vi "iv-sweep-with-dpo3014.vi"(3 "Oscilloscope Address":refnum<visa-resource-name>="USB0::0x0699::0x0411::C023742::INSTR") -> (0 "Indicator of finish":bool=TRUE)   [LabVIEW 2013]
uses:
  <vilib>/Analysis/NI_AALBase.lvlib
  <vilib>/Analysis/baseanly.llb/Mean (DBL).vi
panel:
  in  "Averages":u32=1000 step=1
  out "Channel  1 Graph":dbl[](graph)
  out "Channel  2 Graph":dbl[](graph)
  in  "Cut from end":u32=1000 step=1
  in  "Cut from start":u32=1000 step=1
  in  "Sweep End (V)":dbl=2.0 min=0.002 max=10.0 step=0.001 format="%#_6p"
  in  "Sweep Start (V)":dbl min=0.002 max=10.0 step=0.001 format="%#_6p"
  in  "Sweep Func":u16(ring) items=["SIN", "SQR", "TRI", "RMP", "PLS"]
  in  "Sweep Freq":u16(ring)=15 items=["1MHz", "250kHz", "125kHz", "100kHZ", "25kHz", "10kHz", "5kHz", "2.5kHz", "1kHz", "500Hz", "250Hz", "100Hz", "50Hz", "25Hz", "10Hz", "5Hz", "2.5Hz", "1Hz", "0.5Hz", "0.25Hz"]
  in  "Yokogawa Sweep GPIB":string="18"
  out "Time Range (s)":dbl=0.02 format="%.2p"
  in  "Points per sweep":u16(ring)=1 items=["1000", "10000", "100000", "1000000", "5000000"]
  in  "Trig Delay (s)":dbl step=0.0001 format="%#_6p"
  out "Query Return":string=":ACQUIRE:STOPAFTER SEQUENCE;STATE 1;MODE AVERAGE;NUMENV INFINITE;NUMAVG 2;MAXSAMPLERATE 2.5000E+9\n"
  in  "Query":string="ACQUIRE?"
  out "Time Taken (s)":dbl=1.35 format="%.2p"
  # "If changed, run program once before real readout"
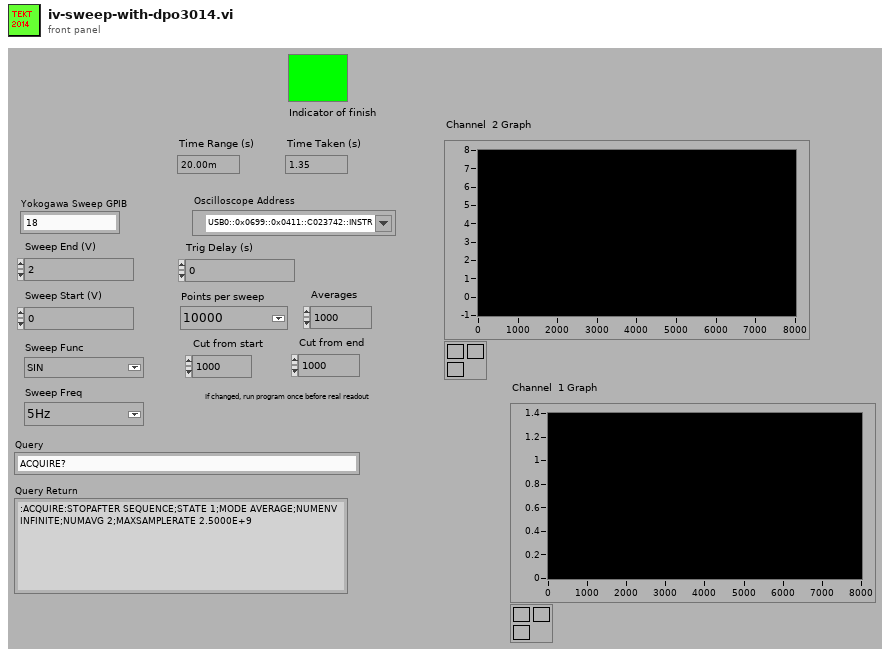
[diagram p1: front panel]
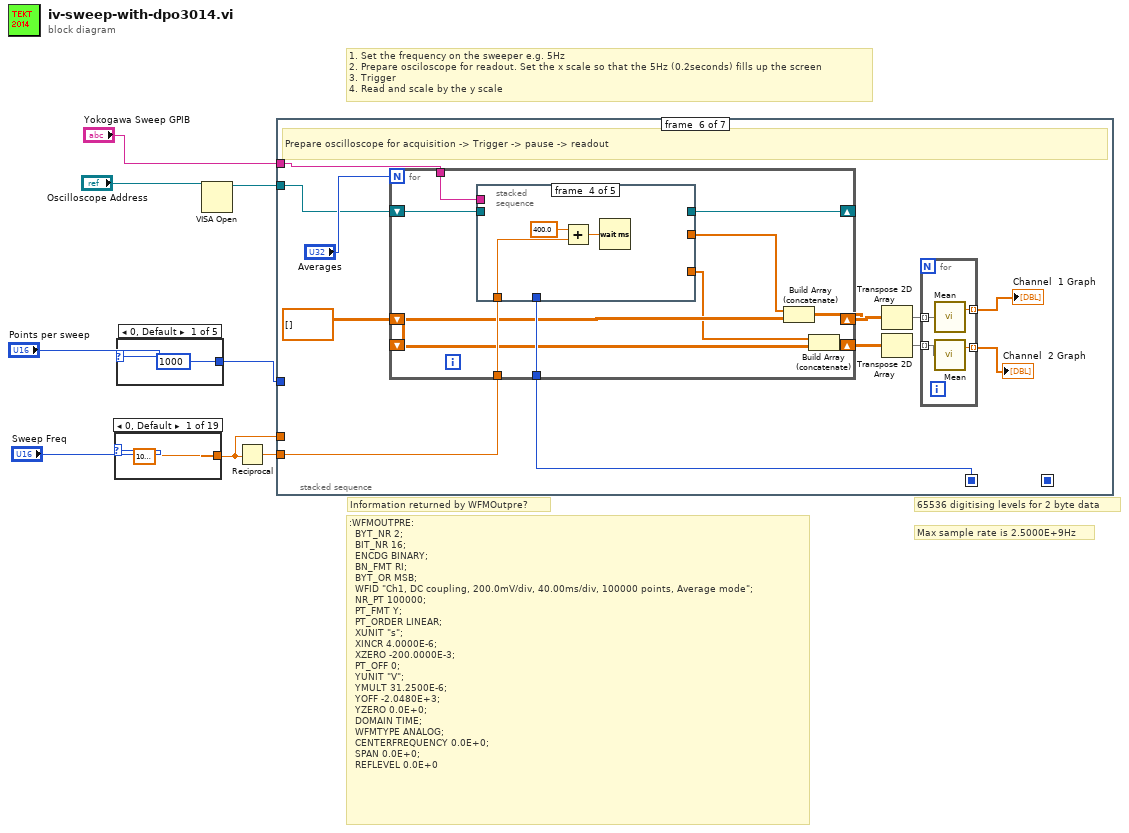
[diagram p0: block diagram]
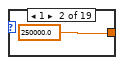
[diagram p2: hidden frame]
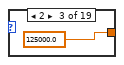
[diagram p3: hidden frame]
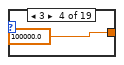
[diagram p4: hidden frame]
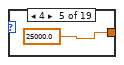
[diagram p5: hidden frame]
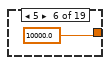
[diagram p6: hidden frame]
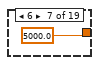
[diagram p7: hidden frame]
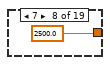
[diagram p8: hidden frame]
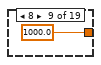
[diagram p9: hidden frame]
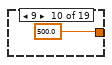
[diagram p10: hidden frame]
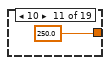
[diagram p11: hidden frame]
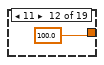
[diagram p12: hidden frame]
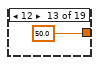
[diagram p13: hidden frame]
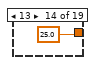
[diagram p14: hidden frame]
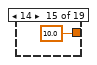
[diagram p15: hidden frame]
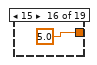
[diagram p16: hidden frame]
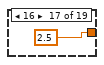
[diagram p17: hidden frame]
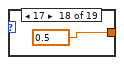
[diagram p18: hidden frame]
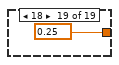
[diagram p19: hidden frame]
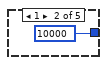
[diagram p20: hidden frame]
diagram:
  # "Max sample rate is 2.5000E+9Hz"
  # "65536 digitising levels for 2 byte data"
  # "Information returned by WFMOutpre?"
  # ":WFMOUTPRE:\n  BYT_NR 2;\n  BIT_NR 16;\n  ENCDG BINARY;\n  BN_FMT RI;\n  BYT_OR MSB;\n  WFID \"Ch1, DC coupling, 200.0mV/div, 40.00ms/div, 100000 points, Average mode\";\n  NR_PT 100000;\n  PT_FMT Y;\n  PT_ORDER LINEAR;\n  XUNIT \"s\";\n  XINCR 4.0000E-6;\n  XZERO -200.0000E-3;\n  PT_OFF 0;\n  YUNIT \"V\";\n  YMULT 31.2500E-6;\n  YOFF -2.0480E+3;\n  YZERO 0.0E+0;\n  DOMAIN TIME;\n  WFMTYPE ANALOG;\n  CENTERFREQUENCY 0.0E+0;\n  SPAN 0.0E+0;\n  REFLEVEL 0.0E+0"
  # "1. Set the frequency on the sweeper e.g. 5Hz\n2. Prepare osciloscope for readout. Set the x scale so that the 5Hz (0.2seconds) fills up the screen\n3. Trigger\n4. Read and scale by the y scale"
  n1 = case shown="0, Default" "Sweep Freq" {
    tunnel: [1000000.0 250000.0 125000.0 100000.0 25000.0 10000.0 5000.0 2500.0 1000.0 500.0 250.0 100.0 50.0 25.0 10.0 5.0 2.5 0.5 0.25] -> w1
    frame 0, Default {
    }
    frame 1 {
    }
    frame 2 {
    }
    frame 3 {
    }
    frame 4 {
    }
    frame 5 {
    }
    frame 6 {
    }
    frame 7 {
    }
    frame 8 {
    }
    frame 9 {
    }
    frame 10 {
    }
    frame 11 {
    }
    frame 12 {
    }
    frame 13 {
    }
    frame 14 {
    }
    frame 15 {
    }
    frame 16 {
    }
    frame 17 {
    }
    frame 18 {
    }
  }
  n2 = case shown="0, Default" "Points per sweep" {
    tunnel: [1000 10000 100000 1000000 5000000] -> w5
    frame 0, Default {
    }
    frame 1 {
    }
    frame 2 {
    }
    frame 3 {
    }
    frame 4 {
    }
  }
  n3 = VISA Open(VISA resource name="Oscilloscope Address") -> (VISA resource name=w7:refnum<visa-resource-name>)  [unwired: 1 in, 4 out]
  n4 = Reciprocal(x=w1) -> (1/x=w4:dbl)
  n5 = stacked-sequence {
    seq-local: [w33 _ _ _ _ _ _] -> [_ _ _ _ _ _ w143]
    seq-local: [_ w35 _ _ _ _ _] -> [_ _ _ _ _ w106 _]
    tunnel: w7 -> [_ w52 _ w86 _ w97 _]
    tunnel: w5 -> [_ w38 _ _ _ _ _]
    tunnel: w4 -> [_ w42 _ _ _ w107 _]
    tunnel: "Yokogawa Sweep GPIB" -> [_ _ w57 _ _ w108 _]
    tunnel: w1 -> [_ _ w74 _ _ _ _]
    frame #0 {
      n6 = Tick Count (ms)() -> (millisecond timer value=w33:u32)
      "Indicator of finish" <- FALSE
    }
    frame #1 {
      # "Number of points\nto read out"
      # "There are 10 divisions on the screen"
      # "Specify which points to return"
      # "- Set number of values to take on the horizontal scale (More datapoints means a higher sample rate)\n- Delay acquisition after trigger\n- Make scale match sweep period"
      # "Specify data type"
      # "Set Paramters on oscilloscope"
      n7 = Divide(x=w42, y=10.0) -> (x/y=w40:dbl)
      "Time Range (s)" <- w40
      n8 = Format Into String(format string=":HORIZONTAL:RECORDLENGTH %d;DELAY:MODE 1;TIME %f;SCALE %f", w38, "Trig Delay (s)", w40) -> (resulting string=w48:string)  [unwired: 2 in, 1 out]
      n9 = VISA Write(VISA resource name=w52, write buffer=":WFMOUTPRE:BYT_NR 2;ENCDG BINARY;BN_FMT RI;BYT_OR MSB;ACQUIRE:NUMAVG 3") -> (VISA resource name out=w49:refnum<visa-resource-name>, error out=w50:errorcluster)  [unwired: 1 in, 1 out]
      n10 = VISA Write(VISA resource name=w49, write buffer=w48, error in (no error)=w50) -> (VISA resource name out=w45:refnum<visa-resource-name>, error out=w44:errorcluster)  [unwired: 1 out]
      n11 = Subtract(x=w38, y="Cut from end") -> (x-y=w37:u32)
      n12 = Subtract(x=w37, y="Cut from start") -> (x-y=w35:u32)
      n13 = Format Into String(format string=":DATA:START %d;STOP %d", "Cut from start", w37) -> (resulting string=w46:string)  [unwired: 2 in, 1 out]
      n14 = VISA Write(VISA resource name=w45, write buffer=w46, error in (no error)=w44) -> ()  [unwired: 3 out]
    }
    frame #2 {
      # "Set parameters on Voltage sweeper"
      n15 = call "span_center_from_min_max.vi"("Begin"="Sweep Start (V)", "End"="Sweep End (V)") -> ("Difference (abs)"=w62:dbl)  [unwired: 1 in, 2 out]
      n16 = Divide(x=w62, y=2.0) -> (x/y=w60:dbl)
      n17 = call "command send GPIB.vi"("Command"="MODE TRIG", "addres"=w57) -> ("error out"=w59:errorcluster)  [unwired: 3 in]
      n18 = Add(x="Sweep Start (V)", y=w60) -> (x+y=w55:dbl)
      n19 = Format Into String(format string="FREQ %f" ("Command"), w74) -> (resulting string=w75:string)  [unwired: 2 in, 1 out]
      n20 = case shown="4" "Sweep Func" {
        tunnel: ["FUNC SIN" ("Command") "FUNC SQR" ("Command") "FUNC TRI" ("Command") "FUNC RMP" ("Command") "FUNC PLS" ("Command")] -> w72
        frame 0, Default {
        }
        frame 1 {
        }
        frame 2 {
        }
        frame 3 {
        }
        frame 4 {
        }
      }
      n21 = Greater?(x=w62, y=1.0) -> (0:w68:bool)
      n22 = call "command send GPIB.vi"("error in"=w59, "Command"=w75, "addres"=w57) -> ("error out"=w58:errorcluster)  [unwired: 2 in]
      n23 = case shown="False" w68 {
        tunnel: ["RANG 1" ("Command") "RANG 10" ("Command")] -> w66
        frame False {
        }
        frame True {
        }
      }
      n24 = call "command send GPIB.vi"("error in"=w58, "Command"=w72, "addres"=w57) -> ("error out"=w71:errorcluster)  [unwired: 2 in]
      n25 = call "command send GPIB.vi"("error in"=w71, "Command"=w66, "addres"=w57) -> ("error out"=w67:errorcluster)  [unwired: 2 in]
      n26 = Format Into String(format string="AMPL %.3f;OFFS %.3f" ("Command"), w62, w55) -> (resulting string=w65:string)  [unwired: 2 in, 1 out]
      n27 = call "command send GPIB.vi"("error in"=w67, "Command"=w65, "addres"=w57) -> ("error out"=w54:errorcluster)  [unwired: 2 in]
      n28 = call "command send GPIB.vi"("error in"=w54, "Command"="CHAN 1;OUTP ON", "addres"=w57) -> ()  [unwired: 2 in, 1 out]
    }
    frame #3 {
      # "Ask for parameters (helps during writting of program)"
      n29 = case shown="False" FALSE {
        tunnel: w86 -> [_ w95]
        frame False {
        }
        frame True {
          # "HEADER 1 will explain returned params"
          n30 = VISA Write(VISA resource name=w95, write buffer="HEADER 1") -> (VISA resource name out=w93:refnum<visa-resource-name>)  [unwired: 1 in, 2 out]
          n31 = VISA Write(VISA resource name=w93, write buffer="Query") -> (VISA resource name out=w94:refnum<visa-resource-name>)  [unwired: 1 in, 2 out]
          n32 = VISA Read(VISA resource name=w94, byte count=u32 2000) -> (VISA resource name out=w88:refnum<visa-resource-name>, read buffer=→"Query Return":string)  [unwired: 1 in, 2 out]
          n33 = VISA Write(VISA resource name=w88, write buffer="HEADER 0") -> ()  [unwired: 1 in, 3 out]
        }
      }
    }
    frame #4 {
      # "Pause for everything to be ready"
      n34 = Wait (ms)(milliseconds to wait=u32 200) -> ()  [unwired: 1 out]
    }
    frame #5 {
      w104 = dbl[][] []
      # "Prepare oscilloscope for acquisition -> Trigger -> pause -> readout"
      n35 = for {
        N: "Averages" -> [_]
        tunnel: w108 -> [w123]
        tunnel: w107 -> [w122]
        tunnel: w106 -> [w121]
        shift-right: [w120] -> w103
        shift-left: w104 -> [w117]
        shift-right: [w114] -> w102
        shift-left: w104 -> [w119]
        shift-right: [w113] -> _
        shift-left: w97 -> [w118]
        n36 = stacked-sequence {
          tunnel: w118 -> [w124 _ _ _ w133]
          tunnel: w123 -> [_ _ w127 _ _]
          tunnel: w122 -> [_ _ _ w129 _]
          tunnel: w121 -> [_ _ _ _ w136]
          tunnel: [_ _ _ _ w135] -> w116
          tunnel: [_ _ _ _ w134] -> w115
          tunnel: [_ _ _ _ w132] -> w113
          frame #0 {
            n37 = VISA Write(VISA resource name=w124, write buffer="ACQ:STATE ON") -> ()  [unwired: 1 in, 3 out]
          }
          frame #1 {
            n38 = Wait (ms)(milliseconds to wait=u32 200) -> ()  [unwired: 1 out]
          }
          frame #2 {
            n39 = call "command send GPIB.vi"("Command"="TRIG", "addres"=w127) -> ()  [unwired: 3 in, 1 out]
          }
          frame #3 {
            n40 = Add(x=400.0 ("y"), y=w129) -> (x+y=w131:dbl)
            n41 = Wait (ms)(milliseconds to wait=w131) -> ()  [unwired: 1 out]
          }
          frame #4 {
            w139 = u16 1 items=["Ch1", "Ch2", "Ch3", "Ch4"] ("Channel")
            w137 = u16 0 items=["Ch1", "Ch2", "Ch3", "Ch4"] ("Channel")
            n42 = call "_dpo3014_read.vi"("Number of points"=w136, "Channel"=w137, "Oscilloscope Address"=w133) -> ("Channel Data"=w134:dbl[], "Oscilloscope Address Out"=w138:refnum<visa-resource-name>)  [unwired: 1 in, 2 out]
            n43 = call "_dpo3014_read.vi"("Number of points"=w136, "Channel"=w139, "Oscilloscope Address"=w138) -> ("Channel Data"=w135:dbl[], "Oscilloscope Address Out"=w132:refnum<visa-resource-name>)  [unwired: 1 in, 2 out]
          }
        }
        n44 = Build Array (concatenate)(w116, w117) -> (w120:dbl[][])
        n45 = Build Array (concatenate)(w115, w119) -> (w114:dbl[][])
      }
      n46 = Transpose 2D Array(2D array=w103) -> (transposed array=w101:dbl[][])
      n47 = Transpose 2D Array(2D array=w102) -> (transposed array=w100:dbl[][])
      n48 = for {
        tunnel: w101 -> [w112] mode=indexing
        tunnel: w100 -> [w110] mode=indexing
        tunnel: [w111] -> w99 mode=indexing
        tunnel: [w109] -> w98 mode=indexing
        n49 = call-poly <vilib>:"Mean.vi"("X"=w112) -> ("mean"=w111:dbl)  [unwired: 1 out]
        n50 = call-poly <vilib>:"Mean.vi"("X"=w110) -> ("mean"=w109:dbl)  [unwired: 1 out]
      }
      "Channel  2 Graph" <- w98
      "Channel  1 Graph" <- w99
    }
    frame #6 {
      n51 = local write "Indicator of finish"(TRUE) -> ()
      n52 = Tick Count (ms)() -> (millisecond timer value=w144:u32)
      n53 = Subtract(x=w144, y=w143) -> (x-y=w142:u32)
      n54 = Divide(x=w142, y=u32 1000) -> (x/y=→"Time Taken (s)":dbl)
    }
  }
